vi "align.vi"(6 "Right-":refnum<vi>, 7 "I2C Ref Out":T1, 8 "error in (no error)":errorcluster, 9 "Right+":refnum<vi>, 10 "Left-":refnum<vi>, 11 "Left+":refnum<vi>) -> (0 "error out":errorcluster, 1 "Aligned":bool, 2 "value Z":ext, 3 "I2C Ref Out out":T1)   [LabVIEW 2017]
uses:
  <vilib>/myRIO/Instrument Drivers/Onboard IO/I2C/typedefs/I2C Reference.ctl
  <vilib>/myRIO/Common/Instrument Driver Framework/Utilities/typedefs/myRIO Generic Hardware Reference.ctl
  <vilib>/myRIO/Common/Instrument Driver Framework/Utilities/typedefs/Hardware Version Enum.ctl
  <vilib>/myRIO/Common/Instrument Driver Framework/Utilities/typedefs/myRIO v1.0 Reference.ctl
  <vilib>/myRIO/Common/Instrument Driver Framework/Utilities/typedefs/Generic FPGA Reference.ctl
  <vilib>/myRIO/Common/Instrument Driver Framework/myRIO v1.0/I2C/typedefs/I2C Channels Enum.ctl
  <vilib>/myRIO/Instrument Drivers/Onboard IO/I2C/typedefs/I2C Configuration.ctl
  <vilib>/myRIO/Instrument Drivers/Onboard IO/I2C/typedefs/I2C Transfer Rate.ctl
  <vilib>/myRIO/Instrument Drivers/Onboard IO/I2C/I2C.lvlib
panel:
  out "offset":ext
  in  "range":ext=5.0 format="%#_13g"
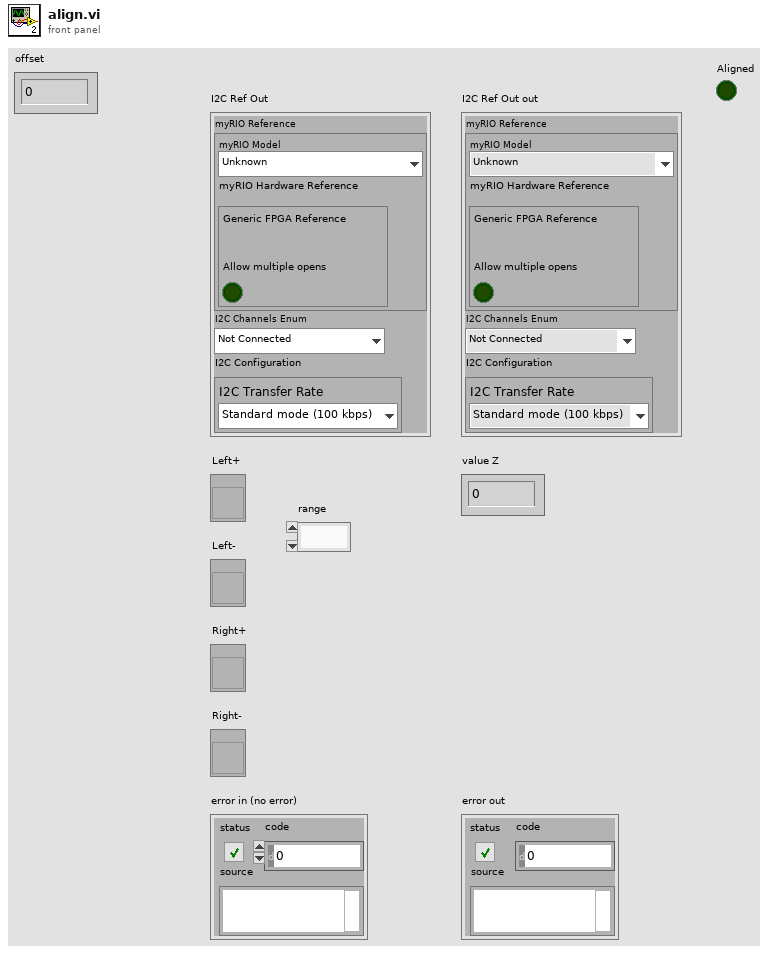
[diagram p1: front panel]
types:
  T1 = typedef "I2C.lvlib/I2C Reference.ctl" = cluster{"myRIO Reference":T2, "I2C Channels Enum":T6, "I2C Configuration":T7}
  T2 = typedef "myRIO Generic Hardware Reference.ctl" = cluster{"myRIO Model":T3, "myRIO Hardware Reference":T4}
  T3 = typedef "Hardware Version Enum.ctl" = enum16{"Unknown", "myRIO-1900", "myRIO-1950", "roboRIO", "NI ELVIS RIO CM"}
  T4 = typedef "myRIO v1.0 Reference.ctl" = cluster{"Generic FPGA Reference":T5, "Allow multiple opens":bool}
  T5 = typedef "Generic FPGA Reference.ctl" = refnum<k20>
  T6 = typedef "I2C Channels Enum.ctl" = enum16{"Not Connected", "A/I2C", "B/I2C", "I2C/I2C"}
  T7 = typedef "I2C.lvlib/I2C Configuration.ctl" = cluster{"I2C Transfer Rate":T8}
  T8 = typedef "I2C.lvlib/I2C Transfer Rate.ctl" = enum16{"Standard mode (100 kbps)", "Fast mode (400 kbps)"}
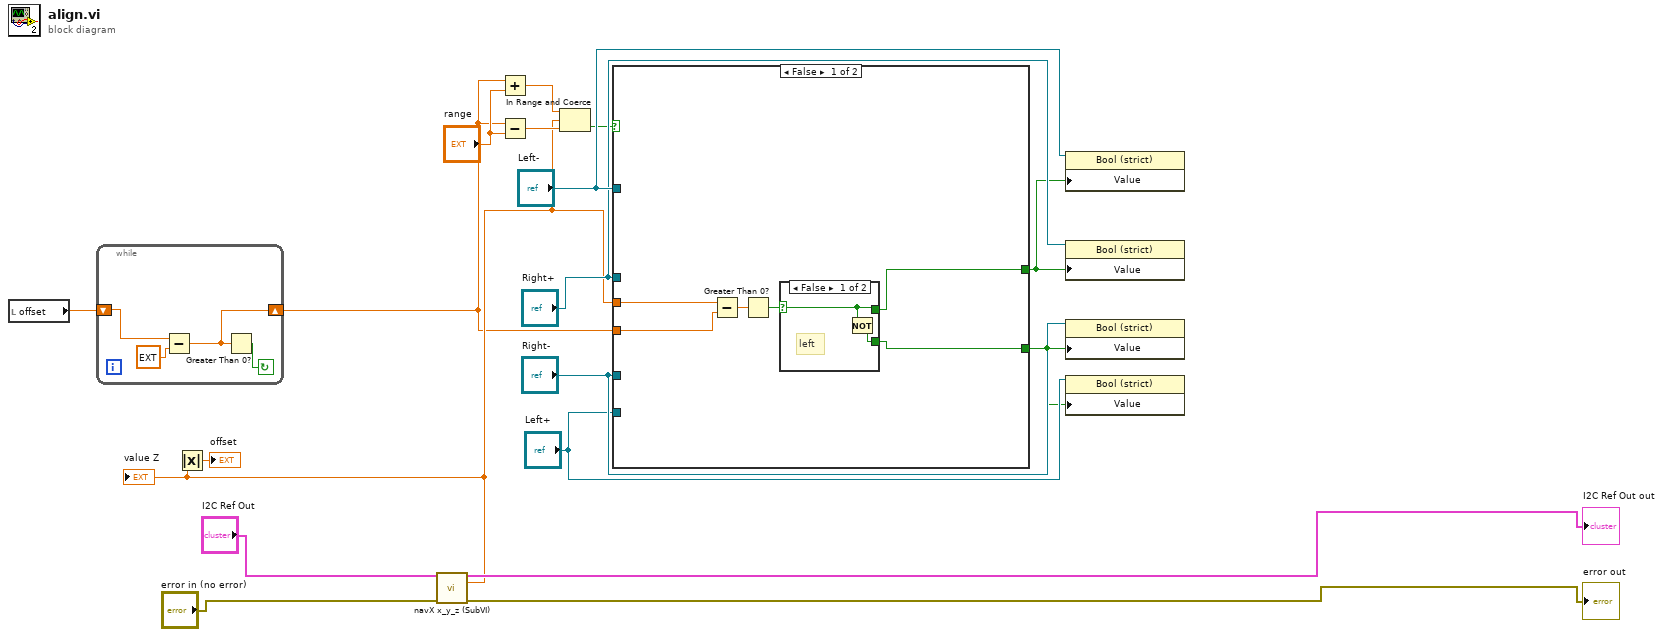
[diagram p0: block diagram]
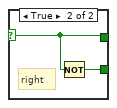
[diagram p2: hidden frame]
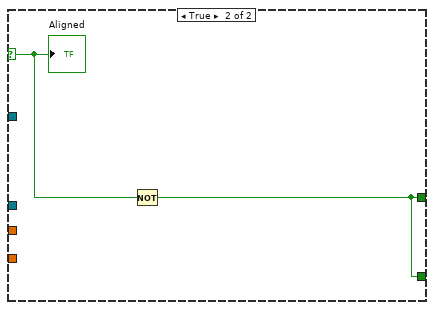
[diagram p3: hidden frame]
diagram:
  n1 = local read "offset"() -> (w3:ext)
  n2 = while {
    shift-right: [w19] -> w1
    shift-left: w3 -> [w20]
    stop <- w21 continue-if-true
    n3 = Subtract(x=w20, y=ext 90.0 ("value Z")) -> (x-y=w19:ext)
    n4 = Greater Than 0?(x=w19) -> (x > 0?=w21:bool)
  }
  n5 = call "navX x_y_z (SubVI).vi"("I2C Ref Out in"="I2C Ref Out", "error in (no error)"="error in (no error)") -> ("I2C Ref Out out"=→"I2C Ref Out out":T1, "value Z"=w4:ext, "error out"=→"error out":errorcluster)  [unwired: 9 in, 2 out]
  "value Z" <- w4
  n6 = Absolute Value(x=w4) -> (abs(x)=→"offset":ext)
  n7 = Add(x=w1, y="range") -> (x+y=w8:ext)
  n8 = Subtract(x=w1, y="range") -> (x-y=w9:ext)
  n9 = In Range and Coerce(upper limit=w8, x=w4, lower limit=w9) -> (In Range?=w7:bool)  [unwired: 1 out]
  n10 = case shown="False" w7 {
    selector: w7 -> [_ w34]
    tunnel: w4 -> [w28 _]
    tunnel: "Left+" -> [_ _]
    tunnel: "Left-" -> [_ _]
    tunnel: "Right+" -> [_ _]
    tunnel: "Right-" -> [_ _]
    tunnel: w1 -> [w25 _]
    tunnel: [w24 w33] -> w5
    tunnel: [w23 w33] -> w6
    frame False {
      n11 = Subtract(x=w28, y=w25) -> (x-y=w26:ext)
      n12 = Greater Than 0?(x=w26) -> (x > 0?=w27:bool)
      n13 = case shown="False" w27 {
        selector: w27 -> [w30 w32]
        tunnel: [w29 w31] -> w24
        tunnel: [w30 w32] -> w23
        frame False {
          # "left"
          n14 = Not(x=w30) -> (.not. x?=w29:bool)
        }
        frame True {
          # "right"
          n15 = Not(x=w32) -> (.not. x?=w31:bool)
        }
      }
    }
    frame True {
      n16 = Not(x=w34) -> (.not. x?=w33:bool)
      "Aligned" <- w34
    }
  }
  n17 = property class="Bool (strict)"(reference="Left-", "Value"=w6) -> ()  [unwired: 1 in, 2 out]
  n18 = property class="Bool (strict)"(reference="Right+", "Value"=w6) -> ()  [unwired: 1 in, 2 out]
  n19 = property class="Bool (strict)"(reference="Right-", "Value"=w5) -> ()  [unwired: 1 in, 2 out]
  n20 = property class="Bool (strict)"(reference="Left+", "Value"=w5) -> ()  [unwired: 1 in, 2 out]
